vi "Ramp Motor Output.vi"(9 "Ramp Time":dbl=250.0 format="%#_13g", 11 "Input":dbl format="%.2f") -> (3 "Output":dbl format="%.2f")   [LabVIEW 2013]
uses:
  Common Code/Change Detect Boolean.vi
  <vilib>/addons/control/pid/pid.llb/PID Output Rate Limiter (DBL).vi
  <vilib>/addons/control/pid/NI_PID_pid.lvlib
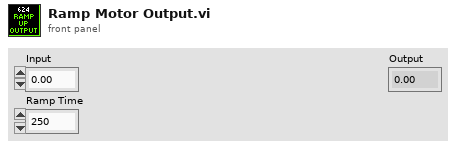
[diagram p1: front panel]
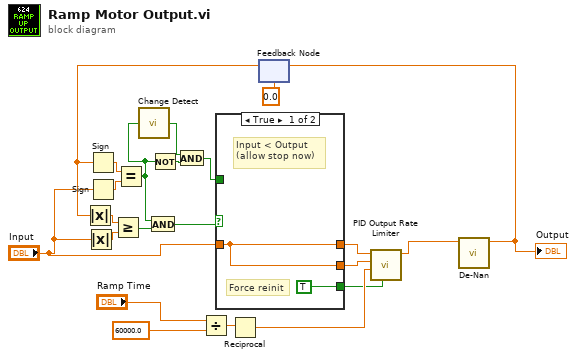
[diagram p0: block diagram]
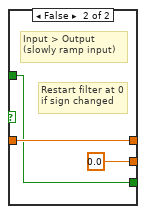
[diagram p2: hidden frame]
diagram:
  n1 = Absolute Value(x="Input") -> (abs(x)=w15:dbl)
  n2 = Sign(1:"Input") -> (0:w12:dbl)
  n3 = Divide(x="Ramp Time", y=60000.0) -> (x/y=w19:dbl)
  n4 = Reciprocal(x=w19) -> (1/x=w18:dbl)
  n5 = feedback #1(0.0 ("initial output")) -> (w10:dbl)
  n6 = Absolute Value(x=w10) -> (abs(x)=w14:dbl)
  n7 = Sign(1:w10) -> (0:w11:dbl)
  n8 = Greater Or Equal?(x=w14, y=w15) -> (x >= y?=w9:bool)
  n9 = Equal?(x=w11, y=w12) -> (x = y?=w5:bool)
  n10 = call-poly "Change Detect.vi"("In"=w5) -> ("Changed?"=w6:bool)
  n11 = And(x=w5, y=w9) -> (x .and. y?=w13:bool)
  n12 = Not(x=w5) -> (.not. x?=w4:bool)
  n13 = And(x=w6, y=w4) -> (x .and. y?=w3:bool)
  n14 = case shown="True" w13 {
    tunnel: [w23 0.0 ("initial output")] -> w22
    tunnel: [TRUE ("reinitialize? (F)") w25] -> w16
    tunnel: "Input" -> [w23 w27]
    tunnel: [w23 w27] -> w8
    tunnel: w3 -> [_ w25]
    frame True {
      # "Force reinit"
      # "Input < Output\n(allow stop now)"
    }
    frame False {
      # "Restart filter at 0\nif sign changed"
      # "Input > Output\n(slowly ramp input)"
    }
  }
  n15 = call-poly <vilib>:"PID Output Rate Limiter.vi"("reinitialize? (F)"=w16, "output rate (EGU/min)"=w18, "initial output"=w22, "input (controller output)"=w8) -> ("output"=w2:dbl)  [unwired: 4 in, 1 out]
  n16 = call "De-Nan.vi"("output in"=w2) -> ("output out"=w1:dbl)  [unwired: 10 in]
  "Output" <- w1
  n17 = feedback-in #1(w1) -> ()
